vi "Set Dac New 3.vi"(0 "DAC nr":u8=1, 1 "DATA (V)":dbl=5000.0 min=-5000.0 max=5000.0 step=0.001 format="%.2f", 2 "error in (no error)":errorcluster) -> (3 "VISA resource name OUT":refnum<visa-resource-name>, 4 "DAC read (mV)":dbl, 5 "DAC nr out":u8, 6 "error out":errorcluster)   [LabVIEW 2011]
uses:
  Visa name1.vi
panel:
  out "DATA (hexadecimaal)":u16=65535 format="%.0x"
  out "DATA (decimaal)":u16=65535
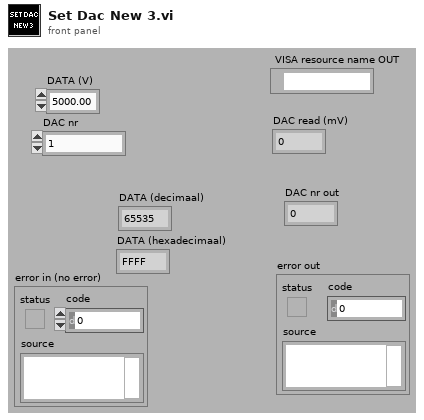
[diagram p1: front panel]
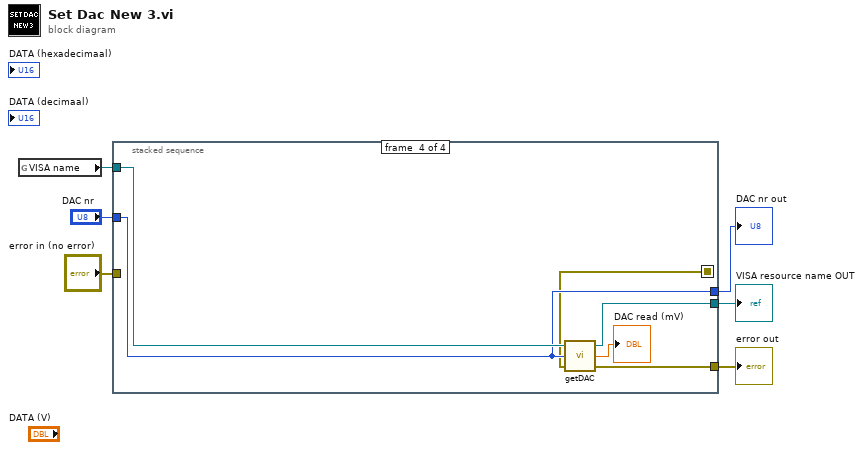
[diagram p0: block diagram]
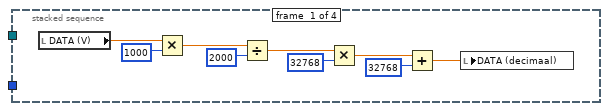
[diagram p2: hidden frame]
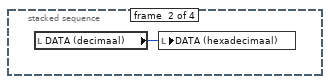
[diagram p3: hidden frame]
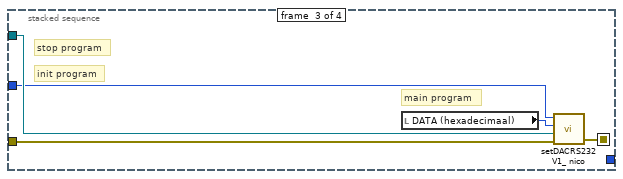
[diagram p4: hidden frame]
diagram:
  n1 = global read "Visa name1.vi" "VISA name"() -> (w3:refnum<visa-resource-name>)
  n2 = stacked-sequence {
    seq-local: [_ _ w17 _] -> [_ _ _ w22]
    tunnel: "error in (no error)" -> [_ _ w20 _]
    tunnel: [_ _ _ w23] -> w5
    tunnel: [_ _ _ w27] -> w4
    tunnel: w3 -> [_ _ w19 w25]
    tunnel: "DAC nr" -> [_ _ w18 w24]
    tunnel: [_ _ _ w24] -> w1
    frame #0 {
      n3 = local read "DATA (V)"() -> (w8:dbl)
      n4 = Multiply(x=w8, y=1000) -> (x*y=w9:dbl)
      n5 = Divide(x=w9, y=2000) -> (x/y=w11:dbl)
      n6 = Multiply(x=w11, y=32768) -> (x*y=w13:dbl)
      n7 = Add(x=w13, y=32768) -> (x+y=w15:dbl)
      n8 = local write "DATA (decimaal)"(w15) -> ()
    }
    frame #1 {
      n9 = local read "DATA (decimaal)"() -> (w16:u16)
      n10 = local write "DATA (hexadecimaal)"(w16) -> ()
    }
    frame #2 {
      # "stop program"
      # "main program"
      # "init program"
      n11 = local read "DATA (hexadecimaal)"() -> (w21:u16)
      n12 = call "setDACRS232 V1_ nico.vi"("error in (no error)"=w20, "VISA resource name IN"=w19, "DATA (hexadecimaal)"=w21, "DAC nr"=w18) -> ("error out"=w17:errorcluster)  [unwired: 1 in, 1 out]
    }
    frame #3 {
      n13 = call "getDAC.vi"("error in (no error)"=w22, "DAC number"=w24, "VISA resource name IN"=w25) -> ("error out"=w23:errorcluster, "DAC read (mV)"=→"DAC read (mV)":dbl, "VISA resource name OUT"=w27:refnum<visa-resource-name>)
    }
  }
  "error out" <- w5
  "VISA resource name OUT" <- w4
  "DAC nr out" <- w1
